vi "HW_GEN - Initialize Current Device Configurations.vi"(8 "error in":errorcluster, 9 "DevInfo[]":T2[](array[typedef]), 10 "HWdef":path, 11 "CFG File":path) -> (0 "error out":errorcluster, 1 "ModuTag[]":string[](array[string]), 2 "sysModCFG[]":T1[](array[typedef]))   [LabVIEW 2016]
doc: "读取配置参数文件，根据硬件信息搜索配置参数是否存在，不存在则创建默认配置参数；\n将新创建的参数保存至配置参数文件中。\n\n针对当前系统的硬件配置生成当前系统的硬件配置信息。"
uses:
  Ctrls/HardWare Basic Info _ Channel.ctl
  Ctrls/HardWare Basic Info _ Module.ctl
  Ctrls/HardWare Basic Info _ Chassis.ctl
  Ctrls/HardWare Basic Info _ Device.ctl
  Ctrls/HardWare _ Module Configuration.ctl
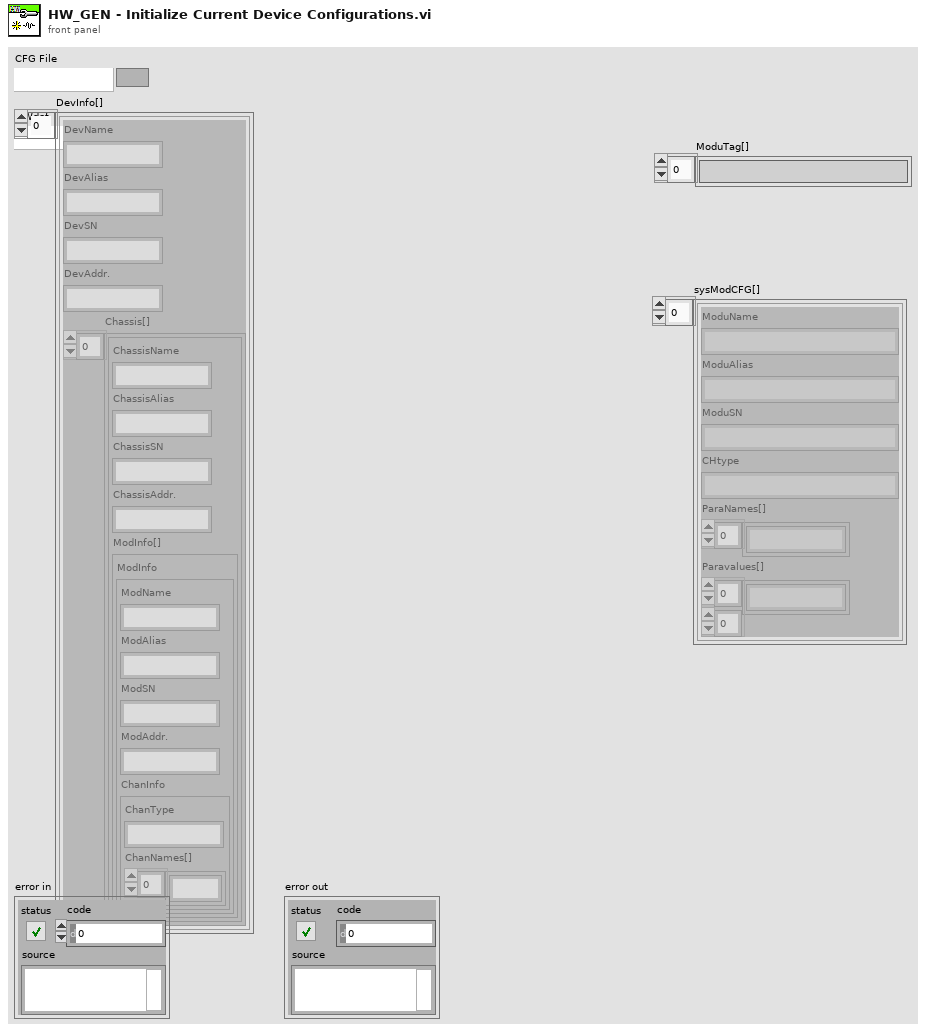
[diagram p1: front panel]
types:
  T1 = typedef "HardWare _ Module Configuration.ctl" = cluster{"ModuName":string, "ModuAlias":string, "ModuSN":string, "CHtype":string, "ParaNames[]":string[], "Paravalues[]":string[][]}
  T2 = typedef "HardWare Basic Info _ Device.ctl" = cluster{"DevName":string, "DevAlias":string, "DevSN":string, "DevAddr.":string, "Chassis[]":T3[]}
  T3 = typedef "HardWare Basic Info _ Chassis.ctl" = cluster{"ChassisName":string, "ChassisAlias":string, "ChassisSN":string, "ChassisAddr.":string, "ModInfo[]":T4[]}
  T4 = typedef "HardWare Basic Info _ Module.ctl" = cluster{"ModName":string, "ModAlias":string, "ModSN":string, "ModAddr.":string, "ChanInfo":T5}
  T5 = typedef "HardWare Basic Info _ Channel.ctl" = cluster{"ChanType":string, "ChanNames[]":string[]}
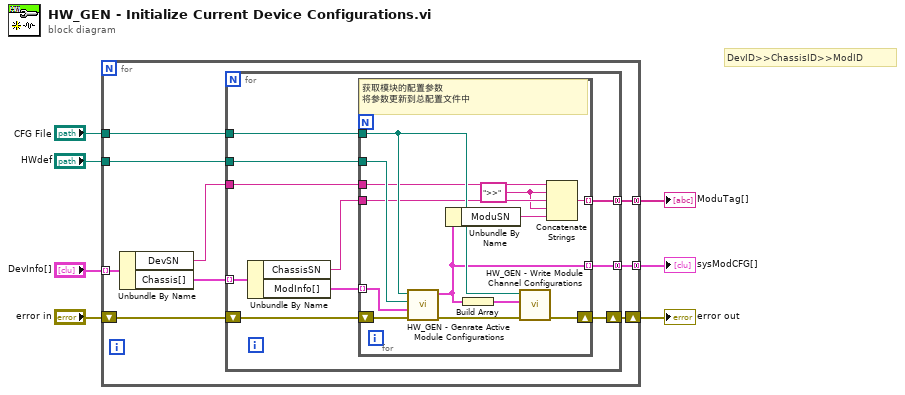
[diagram p0: block diagram]
diagram:
  # "DevID>>ChassisID>>ModID"
  n1 = for {
    shift-right: [w15] -> w4
    shift-left: "error in" -> [w16]
    tunnel: "DevInfo[]" -> [w14] mode=indexing
    tunnel: "CFG File" -> [w13]
    tunnel: "HWdef" -> [w12]
    tunnel: [w10] -> w2 mode=concatenating
    tunnel: [w9] -> w1 mode=concatenating
    n2 = Unbundle By Name(w14) -> ("DevSN"=w8:string, "Chassis[]"=w11:T3[])
    n3 = for {
      shift-right: [w25] -> w15
      shift-left: w16 -> [w26]
      tunnel: w11 -> [w22] mode=indexing
      tunnel: w13 -> [w24]
      tunnel: w12 -> [w23]
      tunnel: [w20] -> w10 mode=concatenating
      tunnel: [w19] -> w9 mode=concatenating
      tunnel: w8 -> [w17]
      n4 = Unbundle By Name(w22) -> ("ChassisSN"=w18:string, "ModInfo[]"=w21:T4[])
      n5 = for {
        tunnel: w24 -> [w35]
        tunnel: w23 -> [w37]
        tunnel: w21 -> [w38] mode=indexing
        shift-right: [w34] -> w25
        shift-left: w26 -> [w39]
        tunnel: [w33] -> w20 mode=indexing
        tunnel: [w28] -> w19 mode=indexing
        tunnel: w18 -> [w31]
        tunnel: w17 -> [w32]
        w30 = ">>" ("string")
        # "获取模块的配置参数\n将参数更新到总配置文件中"
        n6 = call "HW_GEN - Genrate Active Module Configurations.vi"("错误输入"=w39, "ModInfo in"=w38, "HWdef"=w37, "HWcfg Path"=w35) -> ("错误输出"=w36:errorcluster, "ModuCfg"=w33:T1)  [unwired: 5 in, 1 out]
        n7 = Unbundle By Name(w33) -> ("ModuSN"=w29:string)
        n8 = Build Array(w33) -> (w27:T1[])
        n9 = call "HW_GEN - Write Module Channel Configurations.vi"("error in"=w36, "ModCFG.CFG"=w27, "Path"=w35) -> ("error out"=w34:errorcluster)  [unwired: 8 in]
        n10 = Concatenate Strings(w32, w30, w31, w30, w29) -> (w28:string)
      }
    }
  }
  "error out" <- w4
  "sysModCFG[]" <- w2
  "ModuTag[]" <- w1
